vi "Servos-11-15.vi"(0 "Servo2An?":bool, 1 "Servo1An?":bool, 2 "ServosWarmHigh (us)KaltHigh(us)":T1, 3 "ServoTrap2kalt":bool, 4 "ServoTrap1kalt":bool) -> ()   [LabVIEW 2010]
uses:
  <vilib>/eio/EIONode/EIONode.xnode
  <vilib>/rvi/eio/nirviEIOImplementation/nirviEIOImplementation.xnode
  <vilib>/rvi/eio/common/nirviEmuClasses.ctl
  <vilib>/rvi/eio/common/nirviEmuTemplateMethod_noerrors.vi
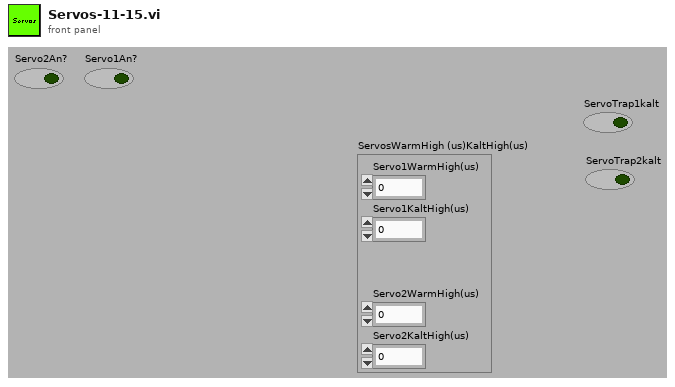
[diagram p1: front panel]
types:
  T1 = cluster{"Servo1WarmHigh(us)":u32, "Servo1KaltHigh(us)":u32, "Servo2WarmHigh(us)":u32, "Servo2KaltHigh(us)":u32}
  T2 = typedef "nirviEmuClasses.ctl" = enum16{"IO Read", "IO Write", "Method", "Property Read", "Property Write"}
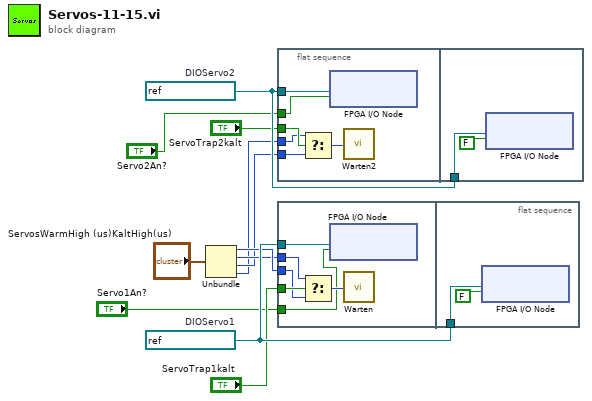
[diagram p0: block diagram]
diagram:
  w11 = refnum<k21> "Mod6/DIO3"  # DIOServo2
  w10 = refnum<k21> "Mod6/DIO2"  # DIOServo1
  n1 = Unbundle("ServosWarmHigh (us)KaltHigh(us)") -> ("Servo1WarmHigh(us)"=w8:u32, "Servo1KaltHigh(us)"=w7:u32, "Servo2WarmHigh(us)"=w6:u32, "Servo2KaltHigh(us)"=w5:u32)
  n2 = flat-sequence {
    tunnel: w11 -> [w17]
    tunnel: "ServoTrap2kalt" -> [w16]
    tunnel: w5 -> [w15]
    tunnel: w6 -> [w14]
    tunnel: "Servo2An?" -> [w12]
    tunnel: w11 -> [w30]
    frame #0 {
      n3 = Select(t=w15, s=w16, f=w14) -> (s? t:f=w13:u32)
      n4 = xnode "FPGA I/O Node"("I/O Item"=w12, "FPGA I/O In"=w17) -> ()  [unwired: 1 out]
      n5 = call "Warten2"("Count(uSec)"=w13) -> ()  [unwired: 1 out]
    }
    frame #1 {
      n6 = xnode "FPGA I/O Node"("I/O Item"=FALSE, "FPGA I/O In"=w30) -> ()  [unwired: 1 out]
    }
  }
  n7 = flat-sequence {
    tunnel: w10 -> [w47]
    tunnel: "ServoTrap1kalt" -> [w46]
    tunnel: w7 -> [w45]
    tunnel: w8 -> [w44]
    tunnel: "Servo1An?" -> [w42]
    tunnel: w10 -> [w60]
    frame #0 {
      n8 = Select(t=w45, s=w46, f=w44) -> (s? t:f=w43:u32)
      n9 = xnode "FPGA I/O Node"("I/O Item"=w42, "FPGA I/O In"=w47) -> ()  [unwired: 1 out]
      n10 = call "Warten"("Count(uSec)"=w43) -> ()  [unwired: 1 out]
    }
    frame #1 {
      n11 = xnode "FPGA I/O Node"("I/O Item"=FALSE, "FPGA I/O In"=w60) -> ()  [unwired: 1 out]
    }
  }
